vi "SetAutoRange.vi"(8 "error in":errorcluster, 10 "Phase":enum16{"OFF", "ON"}(ring), 11 "Port":refnum<visa-resource-name>) -> (0 "error out":errorcluster, 3 "Port out":refnum<visa-resource-name>)   [LabVIEW 2018]
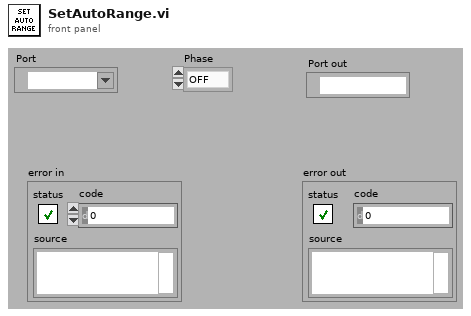
[diagram p1: front panel]
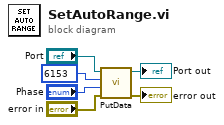
[diagram p0: block diagram]
diagram:
  n1 = call "PutData.vi"("error in"="error in", "Value"="Phase", "Location"=u32 6153, "Port"="Port") -> ("error out"=→"error out":errorcluster, "Port out"=→"Port out":refnum<visa-resource-name>)  [unwired: 6 in]
